vi "to_xml.vi"(8 "error in":errorcluster, 11 "Counter Settings":T1 {"Array of Counter Settings"."Binwidth (ms)" format="%0.2f"}) -> (0 "error out":errorcluster, 3 "counter settings string":string)   [LabVIEW 2013, in "Counter.lvclass"]
doc: "Saves Counter settings to xml in the format:\n\n<Enable>%b</Enable>\n<ArrayOfCounterSettings>\n<counter>\n<CounterChannel>%s</CounterChannel>\n<TimeBinClockChannel>%s</TimeBinClockChannel>\n<binWidth units=\"ms\">%f</binWidth>\n</counter>\n</ArrayOfCounterSettings>\n\nMTL 2013 Jan 1"
uses:
  Counter.lvclass
  Counter_Settings_Control.ctl
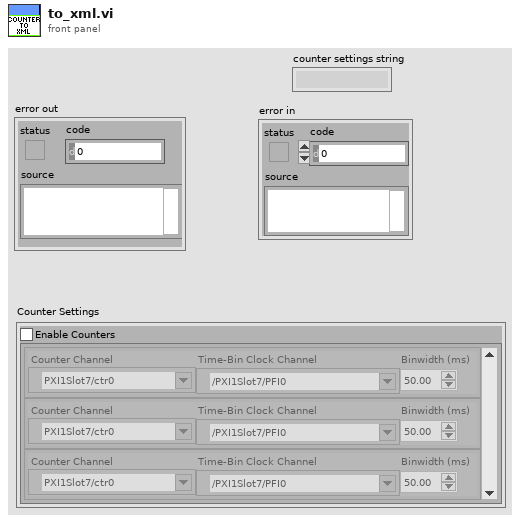
[diagram p1: front panel]
types:
  T1 = typedef "Counter.lvclass/Counter_Settings_Control.ctl" = cluster{"Enable Counters":bool, "Array of Counter Settings":cluster{"Counter Channel":tag, "Time-Bin Clock Channel":tag, "Binwidth (ms)":dbl}[]}
  T2 = cluster{"Counter Channel":tag, "Time-Bin Clock Channel":tag, "Binwidth (ms)":dbl}[]
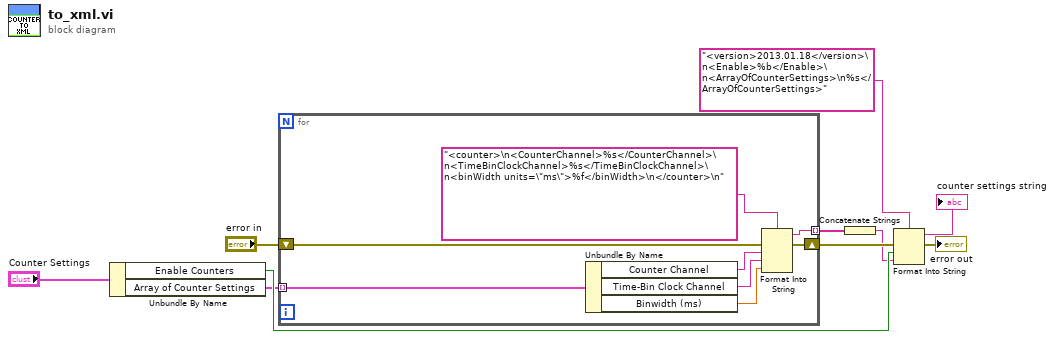
[diagram p0: block diagram]
diagram:
  n1 = Unbundle By Name("Counter Settings") -> ("Enable Counters"=w8:bool, "Array of Counter Settings"=w6:T2)
  n2 = for {
    tunnel: w6 -> [w18] mode=indexing
    shift-right: [w13] -> w4
    shift-left: "error in" -> [w12]
    tunnel: [w11] -> w3 mode=indexing
    n3 = Unbundle By Name(w18) -> ("Counter Channel"=w17:tag, "Time-Bin Clock Channel"=w16:tag, "Binwidth (ms)"=w15:dbl)
    n4 = Format Into String(format string="<counter>\n<CounterChannel>%s</CounterChannel>\n<TimeBinClockChannel>%s</TimeBinClockChannel>\n<binWidth units=\"ms\">%f</binWidth>\n</counter>\n", error in=w12, w17, w16, w15) -> (resulting string=w11:string, error out=w13:errorcluster)  [unwired: 1 in]
  }
  n5 = Concatenate Strings(w3) -> (w2:string)
  n6 = Format Into String(format string="<version>2013.01.18</version>\n<Enable>%b</Enable>\n<ArrayOfCounterSettings>\n%s</ArrayOfCounterSettings>", error in=w4, w8, w2) -> (resulting string=→"counter settings string":string, error out=→"error out":errorcluster)  [unwired: 1 in]
